vi "PH_Tektronix_7000.contents.vi"   [LabVIEW 2014, in "PH_Tektronix_7000.lvlib"]
doc: "This class is forseen to xxx\n\nThis class is part of the PHELIX xxx layer."
uses:
  PH_Tektronix_7000.lvlib
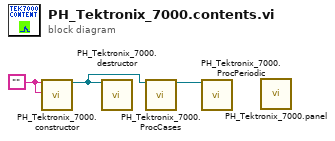
[diagram p0: block diagram]
diagram:
  w2 = ""
  n1 = call "PH_Tektronix_7000.constructor.vi"("name"=w2, "data in"=w2) -> ("i ref out"=w1:refnum<vi>)  [unwired: 15 in, 2 out]
  n2 = call "PH_Tektronix_7000.destructor.vi"("i ref in"=w1) -> ()  [unwired: 18 in, 1 out]
  n3 = call "PH_Tektronix_7000.ProcCases.vi"("i ref in"=w1) -> ("i ref out"=w3:refnum<vi>)  [unwired: 16 in, 2 out]
  n4 = call "PH_Tektronix_7000.ProcPeriodic.vi"("i ref in"=w3) -> ()  [unwired: 16 in, 3 out]
  n5 = call "PH_Tektronix_7000.panel.vi"() -> ()  [unwired: 19 in, 1 out]
